vi "Parse Monitor Result.vi"(8 "Boolean In":bool, 11 "Node Id In":string) -> (0 "Value Out":bool, 3 "element":string)   [LabVIEW 2024]
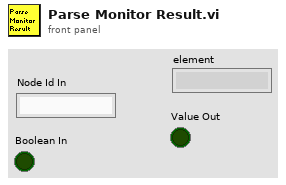
[diagram p1: front panel]
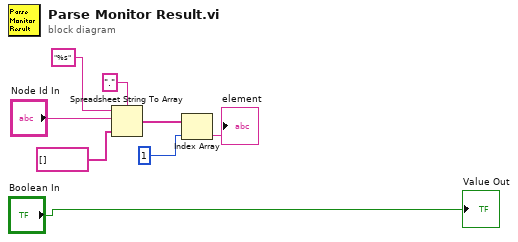
[diagram p0: block diagram]
diagram:
  n1 = Spreadsheet String To Array(delimiter (Tab)=".", format string="%s", spreadsheet string="Node Id In", array type (2D Dbl)=string[] []) -> (array=w4:string[])
  n2 = Index Array(array=w4, index=1) -> (element=→"element":string)
  "Value Out" <- "Boolean In"
